vi "Client.vi"() -> ()   [LabVIEW 2020]
uses:
  <vilib>/event_ctls.llb/eventvkey.ctl
  <userlib>/_NEVSTOP/Communicable State Machine(CSM)/AdvanceAPI/CSM - Keywords.vi
  <userlib>/_NEVSTOP/Communicable State Machine(CSM)/_Support/Common/Trim Single line Text.vi
  <userlib>/_NEVSTOP/GlobalStop/_gStop.vi
  <userlib>/_NEVSTOP/GlobalStop/GSTOP.lvlib
  <userlib>/_NEVSTOP/Communicable State Machine(CSM)/Communicable State Machine.lvlib
  <userlib>/_NEVSTOP/Communicable State Machine(CSM)/addons/API-String-Arugments-Support/API String Arguments Support.lvlib
  a1c83761-5f2f-4742-9fa6-a9430ba65f56.vi
panel:
  out "Console":string
  in  "Command":string caption="$"
  out "To Who":string
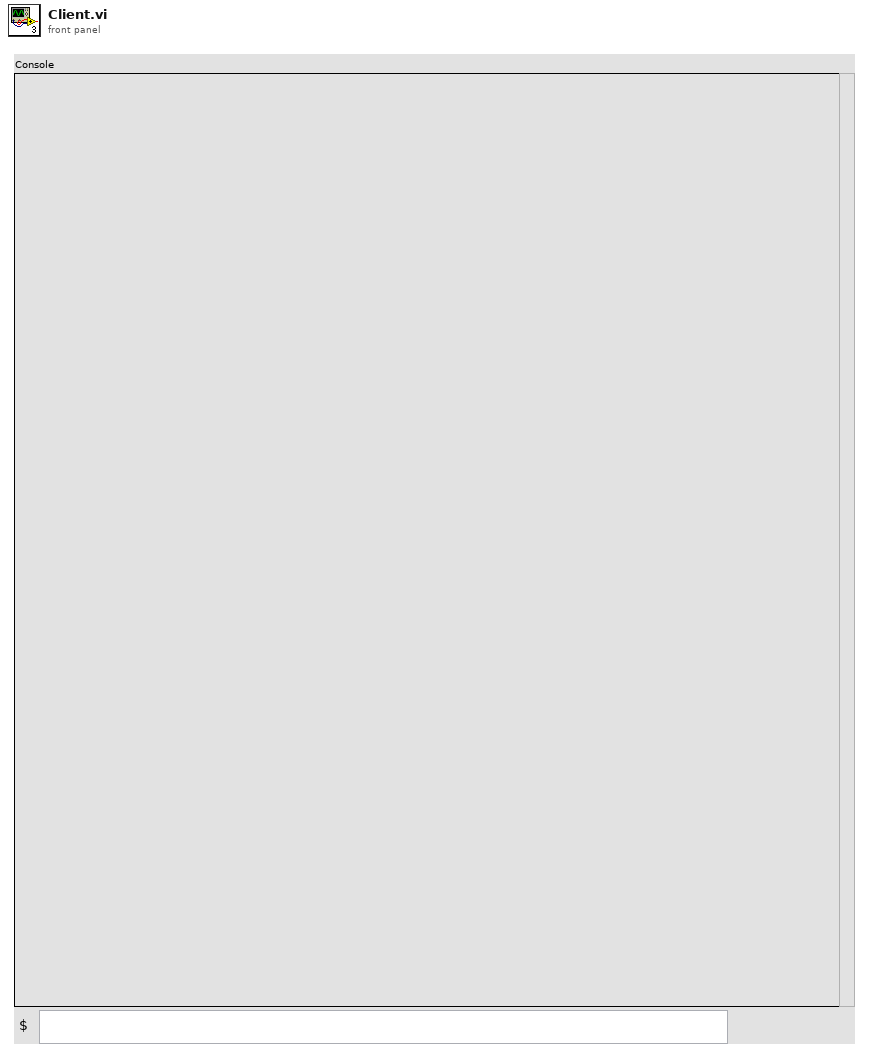
[diagram p1: front panel]
types:
  T1 = typedef "eventvkey.ctl" = enum16{"ASCII", "Enter", "Return", "Shift", "Ctrl", "Alt", "Cmd", "Opt", "Caps", "NumLock", "Clear", "Break", "Up", "Down", "Left", "Right", "Insert", "Delete", "Home", "End", "PageUp", "PageDown", "Escape", "Help", "Pause", "ScrollLock", "F1", "F2", "F3", "F4", "F5", "F6", "F7", "F8", "F9", "F10", "F11", "F12", "F13", "F14", "F15", "F16", "F17", "F18", "F19", "F20", "F21", "F22", "F23", "F24", "Play", "VolumeUp", "VolumeDown", "Mute", "Two Byte Char"}
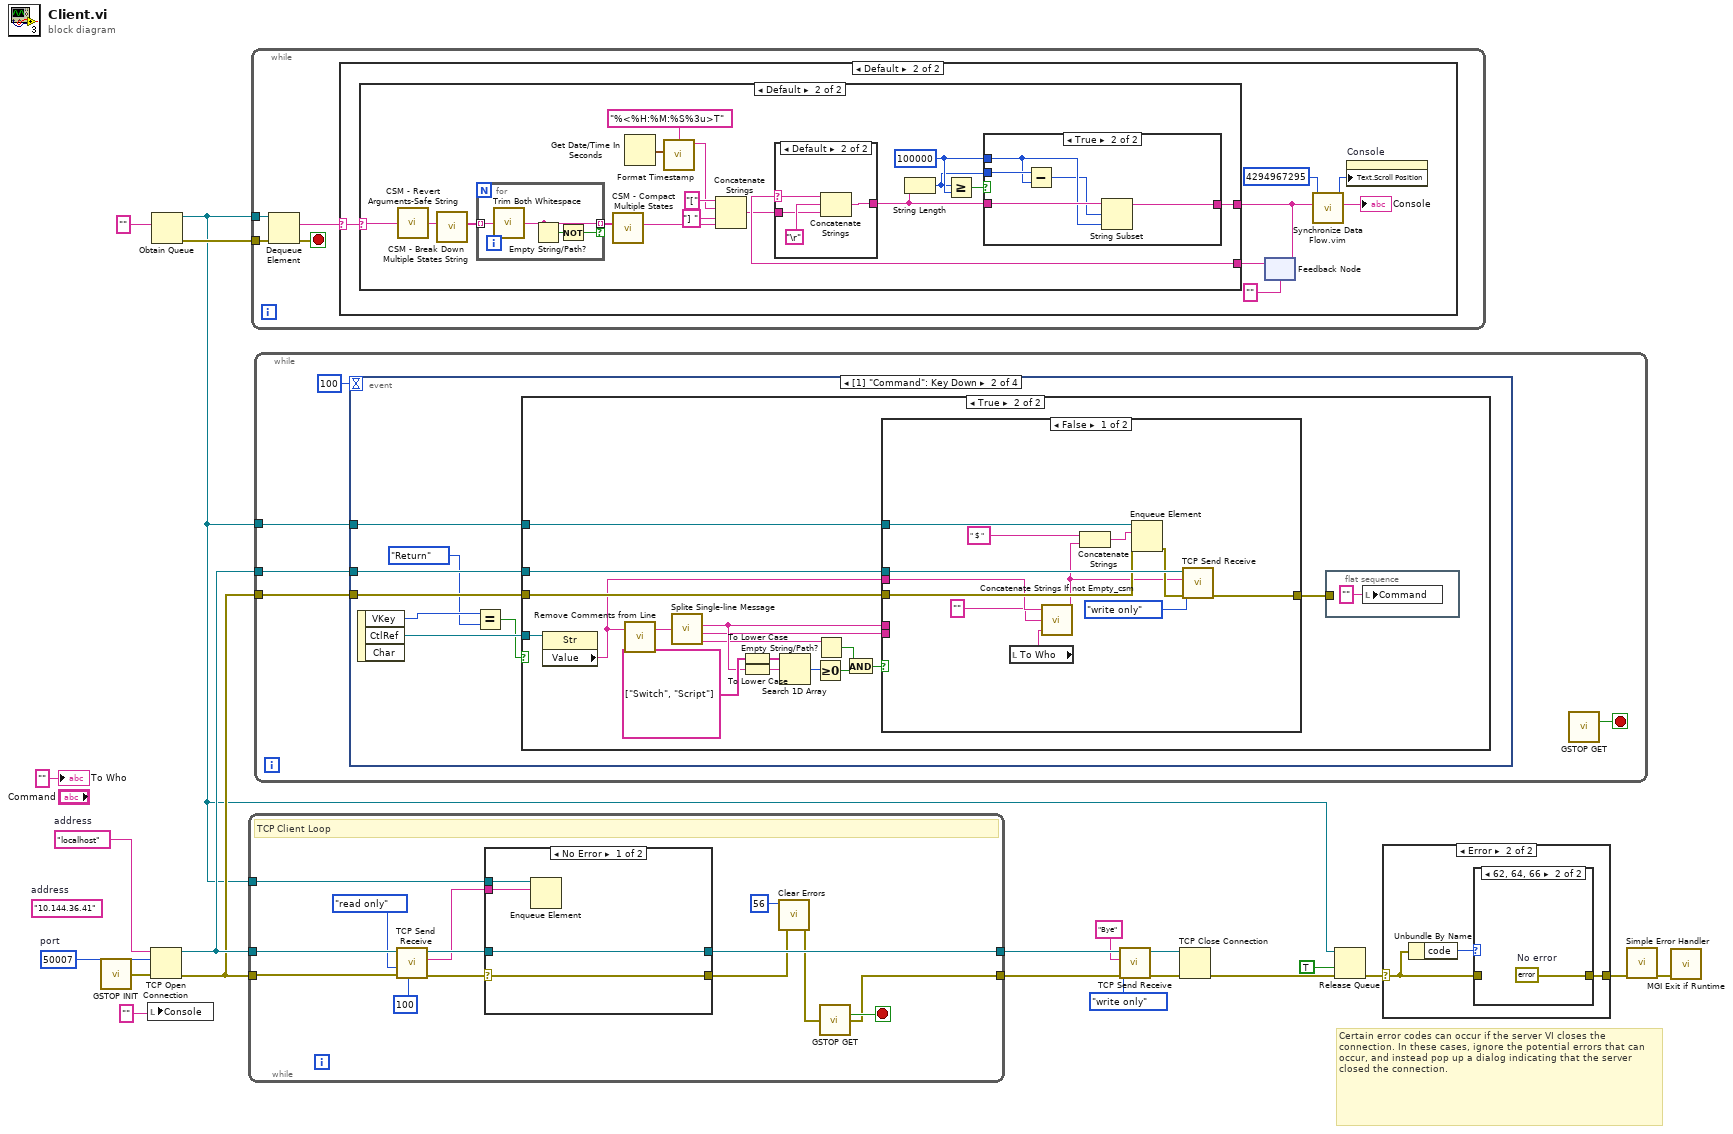
[diagram p0: block diagram]
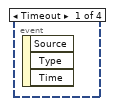
[diagram p6: hidden frame]
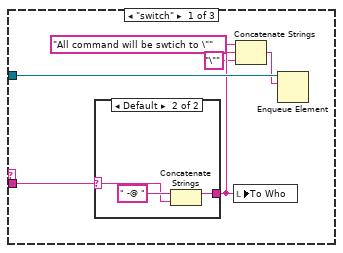
[diagram p9: hidden frame]
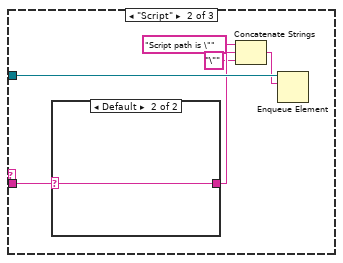
[diagram p11: hidden frame]
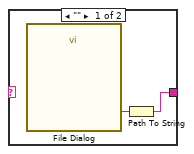
[diagram p12: hidden frame]
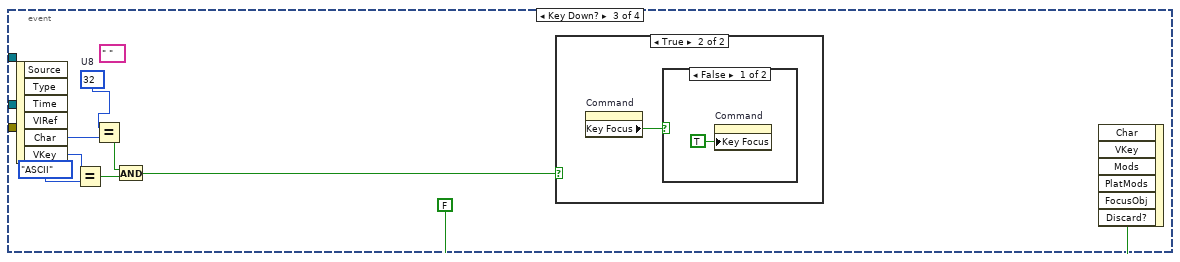
[diagram p13: hidden frame]
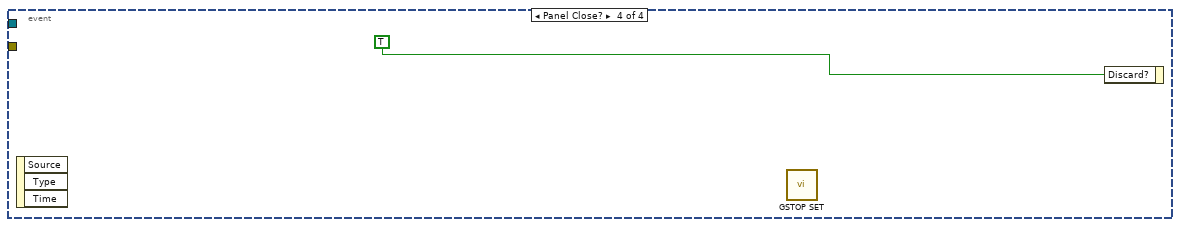
[diagram p16: hidden frame]
diagram:
  w2 = "localhost"  # address
  w15 = u16 50007  # port
  (unwired) "10.144.36.41"  # address
  # "Certain error codes can occur if the server VI closes the connection. In these cases, ignore the potential errors that can occur, and instead pop up a dialog indicating that the server closed the connection."
  n1 = call <userlib>:"GSTOP INIT.vi"() -> ("error out"=w11:errorcluster)  [unwired: 15 in]
  n2 = local write "Console"("" ("data out")) -> ()
  n3 = TCP Open Connection(address=w2, remote port or service name=w15, error in (no error)=w11) -> (connection ID=w13:refnum<k5>, error out=w12:errorcluster)  [unwired: 2 in]
  n4 = Obtain Queue(element data type="" ("name (unnamed)")) -> (queue out=w5:refnum<queue>, error out=w9:errorcluster)  [unwired: 4 in, 1 out]
  n5 = while {
    tunnel: w12 -> [w32]
    tunnel: w13 -> [w33]
    tunnel: [w31] -> w20
    tunnel: [w22] -> w18
    tunnel: w5 -> [w24]
    stop <- w26 stop-if-true
    # "TCP Client Loop"
    n6 = call "TCP Send Receive.vi"("timeout ms (1000)"=100, "error in (no error)"=w32, "access (read/write)"=enum16{"read/write", "read only", "write only"}."read only", "connection ID"=w33) -> ("error out"=w34:errorcluster, "Data Out"=w27:string, "connection ID Out"=w35:refnum<k5>)  [unwired: 5 in]
    n7 = case shown="No Error" w34 {
      selector: w34 -> [w38 w41]
      tunnel: w35 -> [w39 w40]
      tunnel: [w39 w40] -> w31
      tunnel: [w38 w41] -> w30
      tunnel: w27 -> [w36 _]
      tunnel: w24 -> [w37 _]
      frame No Error {
        n8 = Enqueue Element(queue=w37, element=w36) -> ()  [unwired: 2 in, 3 out]
      }
      frame Error {
      }
    }
    n9 = call <vilib>:"Clear Errors.vi"("error in (no error)"=w30, "specific error code to clear (0: all)"=56) -> ("error out"=w23:errorcluster)  [unwired: 4 in, 1 out]
    n10 = call <userlib>:"GSTOP GET.vi"("error in (no error)"=w23) -> ("stop"=w26:bool, "error out"=w22:errorcluster)  [unwired: 13 in]
  }
  n11 = while {
    tunnel: w9 -> [w44]
    tunnel: w5 -> [w45]
    stop <- w43 stop-if-true
    n12 = Dequeue Element(queue=w45, error in (no error)=w44) -> (element=w42:string, error out=w43:errorcluster)  [unwired: 1 in, 2 out]
    n13 = case shown="Default" w42 {
      selector: w42 -> [_ w49]
      frame "" {
      }
      frame Default {
        n14 = feedback #1("") -> (w52:string)
        n15 = case shown="Default" w49 {
          selector: w49 -> [_ w55]
          tunnel: w52 -> [w53 w67]
          tunnel: [w53 w70] -> w50
          frame "" {
          }
          frame Default {
            w64 = 100000 ("length")
            n16 = call <userlib>:"CSM - Revert Arguments-Safe String.vi"("Safe Argurment String"=w55) -> ("Origin Argurment String"=w57:string)  [unwired: 8 in]
            n17 = call <userlib>:"CSM - Break Down Multiple States String.vi"("States"=w57) -> ("Multiple States"=w56:string[])  [unwired: 10 in]
            n18 = for {
              tunnel: w56 -> [w74] mode=indexing
              tunnel: [w73] -> w58 mode=indexing if=w71
              n19 = call <userlib>:"Trim Both Whitespace.vi"("string"=w74) -> ("trimmed string"=w73:string)  [unwired: 1 in]
              n20 = Empty String/Path?(string/path=w73) -> (empty?=w72:bool)
              n21 = Not(x=w72) -> (.not. x?=w71:bool)
            }
            n22 = call <userlib>:"CSM - Compact Multiple States.vi"("Multiple States"=w58) -> ("States"=w54:string)  [unwired: 9 in]
            n23 = Get Date/Time In Seconds() -> (seconds since 1Jan1904=w59:timestamp)
            n24 = call <userlib>:"Format Timestamp.vi"("timestamp"=w59, "format string"="%<%H:%M:%S%3u>T") -> ("String"=w61:string)  [unwired: 9 in]
            n25 = Concatenate Strings("[" ("string"), w61, "] " ("string"), w54) -> (w66:string)
            n26 = case shown="Default" w67 {
              selector: w67 -> [_ w83]
              tunnel: [w81 w84] -> w65
              tunnel: w66 -> [w81 w82]
              frame "" {
              }
              frame Default {
                n27 = Concatenate Strings(w83, "\r", w82) -> (w84:string)
              }
            }
            n28 = String Length(string=w65) -> (length=w62:i32)
            n29 = Greater Or Equal?(x=w62, y=w64) -> (x >= y?=w63:bool)
            n30 = case shown="True" w63 {
              tunnel: [w75 w80] -> w70
              tunnel: w65 -> [w75 w79]
              tunnel: w64 -> [_ w77]
              tunnel: w62 -> [_ w78]
              frame False {
              }
              frame True {
                n31 = Subtract(x=w78, y=w77) -> (x-y=w76:i32)
                n32 = String Subset(string=w79, offset (0)=w76, length (rest)=w77) -> (substring=w80:string)
              }
            }
          }
        }
        n33 = feedback-in #1(w50) -> ()
        n34 = call "Synchronize Data Flow.vim"("input 2"=w50, "input 1"=u32 4294967295 ("Text.Scroll Position")) -> ("output 2"=→"Console":string, "output 1"=w46:u32)  [unwired: 2 in, 2 out]
        n35 = property on="Console" class="Str"("Text.Scroll Position"=w46) -> ()  [unwired: 2 in, 2 out]
      }
    }
  }
  n36 = while {
    tunnel: w13 -> [w90]
    tunnel: w12 -> [w89]
    tunnel: w5 -> [w87]
    stop <- w86 stop-if-true
    n37 = event shown="[1] \"Command\": Key Down" {
      selector: _ -> [_ _ _ _]
      dyn-events: _ -> [_ _ _ _]
      timeout: 100 -> [_ _ _ _]
      tunnel: w90 -> [_ w97 _ _]
      tunnel: w89 -> [_ w95 _ _]
      tunnel: w87 -> [_ w96 _ _]
      event Timeout {
        n38 = event-data() -> ()  [unwired: 1 in, 3 out]
      }
      event "Command": Key Down {
        n39 = event-data() -> ("VKey"=w93:T1, "CtlRef"=w94:refnum<vi>)  [unwired: 1 in, 1 out]
        n40 = Equal?(x=w93, y=eventvkey."Return") -> (x = y?=w91:bool)
        n41 = case shown="True" w91 {
          tunnel: w97 -> [_ w114]
          tunnel: w96 -> [_ w113]
          tunnel: w95 -> [_ w112]
          tunnel: w94 -> [_ w111]
          frame False {
          }
          frame True {
            n42 = property class="Str"(reference=w111) -> ("Value"=w108:string)  [unwired: 1 in, 2 out]
            n43 = call <userlib>:"Remove Comments from Line.vi"("single-line text"=w108) -> ("single-line text without comments"=w109:string)  [unwired: 2 in]
            n44 = call <userlib>:"Splite Single-line Message.vi"("single-line text"=w109) -> ("state"=w106:string, "args"=w98:string, "source/target"=w99:string)  [unwired: 6 in, 1 out]
            n45 = To Lower Case(string=string[] ["Switch", "Script"] ("hostname")) -> (all lower case string=w101:string[])
            n46 = To Lower Case(string=w106) -> (all lower case string=w100:string)
            n47 = Search 1D Array(1D array=w101, element=w100) -> (index of element=w105:i32)  [unwired: 1 in]
            n48 = Greater Or Equal To 0?(x=w105) -> (x >= 0?=w104:bool)
            n49 = Empty String/Path?(string/path=w99) -> (empty?=w103:bool)
            n50 = And(x=w103, y=w104) -> (x .and. y?=w102:bool)
            n51 = case shown="False" w102 {
              tunnel: w114 -> [w125 _]
              tunnel: w113 -> [w124 w129]
              tunnel: w112 -> [w120 w130]
              tunnel: [w119 w130] -> w110
              tunnel: w108 -> [w118 _]
              tunnel: w106 -> [_ w127]
              tunnel: w98 -> [_ w128]
              frame False {
                n52 = local read "To Who"() -> (w115:string)
                n53 = call <userlib>:"Concatenate Strings If not Empty_csm.vi"("String"=w115, "seperator(:)"="", "prefix"=w118) -> ("result"=w117:string)  [unwired: 2 in]
                n54 = Concatenate Strings(" $ " ("string"), w117) -> (w122:string)
                n55 = Enqueue Element(queue=w124, element=w122, error in (no error)=w120) -> (error out=w121:errorcluster)  [unwired: 1 in, 2 out]
                n56 = call "TCP Send Receive.vi"("error in (no error)"=w121, "access (read/write)"=enum16{"read/write", "read only", "write only"}."write only", "Data In"=w117, "connection ID"=w125) -> ("error out"=w119:errorcluster)  [unwired: 5 in, 2 out]
              }
              frame True {
                n57 = case shown="Default" w127 {
                  tunnel: w129 -> [w135 w144 _]
                  tunnel: w128 -> [w136 w145 _]
                  frame "switch" {
                    n58 = case shown="Default" w136 {
                      selector: w136 -> [_ w137]
                      tunnel: [_ w138] -> w134
                      frame "" {
                      }
                      frame Default {
                        n59 = Concatenate Strings(" -@ " ("To Who"), w137) -> (w138:string)
                      }
                    }
                    n60 = local write "To Who"(w134) -> ()
                    n61 = Concatenate Strings("All command will be swtich to \"" ("string"), w134, "\"" ("string")) -> (w133:string)
                    n62 = Enqueue Element(queue=w135, element=w133) -> ()  [unwired: 2 in, 3 out]
                  }
                  frame "Script" {
                    n63 = case shown="Default" w145 {
                      selector: w145 -> [_ w148]
                      tunnel: [w146 w148] -> w143
                      frame "" {
                        n64 = call "File Dialog"() -> ("selected path"=w147:path)  [unwired: 12 in, 3 out]
                        n65 = Path To String(path=w147) -> (string=w146:string)
                      }
                      frame Default {
                      }
                    }
                    n66 = Concatenate Strings("Script path is \"" ("string"), w143, "\"" ("string")) -> (w142:string)
                    n67 = Enqueue Element(queue=w144, element=w142) -> ()  [unwired: 2 in, 3 out]
                  }
                  frame Default {
                  }
                }
              }
            }
            n68 = flat-sequence {
              tunnel: w110 -> [_]
              frame #0 {
                n69 = local write "Command"("" ("Command")) -> ()
              }
            }
          }
        }
      }
      event Key Down? {
        (unwired) " "
        w152 = u8 32  # U8
        n70 = event-data() -> ("Char"=w153:i16, "VKey"=w155:T1)  [unwired: 1 in, 4 out]
        n71 = Equal?(x=w155, y=eventvkey."ASCII" ("VKey")) -> (x = y?=w154:bool)
        n72 = Equal?(x=w152, y=w153) -> (x = y?=w151:bool)
        n73 = And(x=w151, y=w154) -> (x .and. y?=w150:bool)
        n74 = case shown="True" w150 {
          frame False {
          }
          frame True {
            n75 = property on="Command" class="Str"() -> ("Key Focus"=w158:bool)  [unwired: 2 in, 2 out]
            n76 = case shown="False" w158 {
              frame False {
                n77 = property on="Command" class="Str"("Key Focus"=TRUE) -> ()  [unwired: 2 in, 2 out]
              }
              frame True {
              }
            }
          }
        }
        n78 = event-data("Discard?"=FALSE) -> ()  [unwired: 6 in, 1 out]
      }
      event Panel Close? {
        n79 = event-data() -> ()  [unwired: 1 in, 3 out]
        n80 = call <userlib>:"GSTOP SET.vi"() -> ()  [unwired: 15 in, 1 out]
        n81 = event-data("Discard?"=TRUE) -> ()  [unwired: 1 in, 1 out]
      }
    }
    n82 = call <userlib>:"GSTOP GET.vi"() -> ("stop"=w86:bool)  [unwired: 14 in, 1 out]
  }
  n83 = call "TCP Send Receive.vi"("error in (no error)"=w18, "access (read/write)"=enum16{"read/write", "read only", "write only"}."write only", "Data In"="Bye", "connection ID"=w20) -> ("error out"=w19:errorcluster, "connection ID Out"=w21:refnum<k5>)  [unwired: 5 in, 1 out]
  n84 = TCP Close Connection(connection ID=w21, error in (no error)=w19) -> (error out=w7:errorcluster)  [unwired: 1 in, 1 out]
  n85 = Release Queue(queue=w5, force destroy? (F)=TRUE, error in (no error)=w7) -> (error out=w6:errorcluster)  [unwired: 2 out]
  n86 = case shown="Error" w6 {
    selector: w6 -> [w161 w163]
    tunnel: [w161 w162] -> w16
    frame No Error {
    }
    frame Error {
      n87 = Unbundle By Name(w163) -> ("code"=w164:i32)
      n88 = case shown="62, 64, 66" w164 {
        tunnel: w163 -> [w165 _]
        tunnel: [w165 w166] -> w162
        frame Default {
        }
        frame 62, 64, 66 {
          w166 = errorcluster {"status"=FALSE, "code"=0, "source"=""}  # No error
        }
      }
    }
  }
  n89 = call <vilib>:"Simple Error Handler.vi"("error in (no error)"=w16) -> ("error out"=w1:errorcluster)  [unwired: 4 in, 4 out]
  n90 = call <userlib>:"MGI Exit if Runtime.vi"("Error In (Dependency Only)"=w1) -> ()  [unwired: 11 in]
  "To Who" <- "" ("hostname")
